vi "从数据库获取数据通用可配置(子VI).vi"(8 "错误输入（无错误）":errorcluster, 9 "查询参数数组":string[](array[string])=["CODMn", "CODCr", "DO", "铜", "PH", "氨氮", "比电导率", "水温", "COD", "浊度", "总氮", "总磷", "叶绿素a", "藻密度", "水位", "流速", "瞬时流量", "累积流量", "亚硝酸盐", "硫化物", "ORP", "铅", "镉", "锌", "镍", "锰", "汞"], 10 "table输入":string="实时数据") -> (0 "错误输出":errorcluster, 3 "簇数组":cluster{"待发送数据":string[][]}[][](array[cluster]))   [LabVIEW 2016, in "数据传输系统-02.lvlib"]
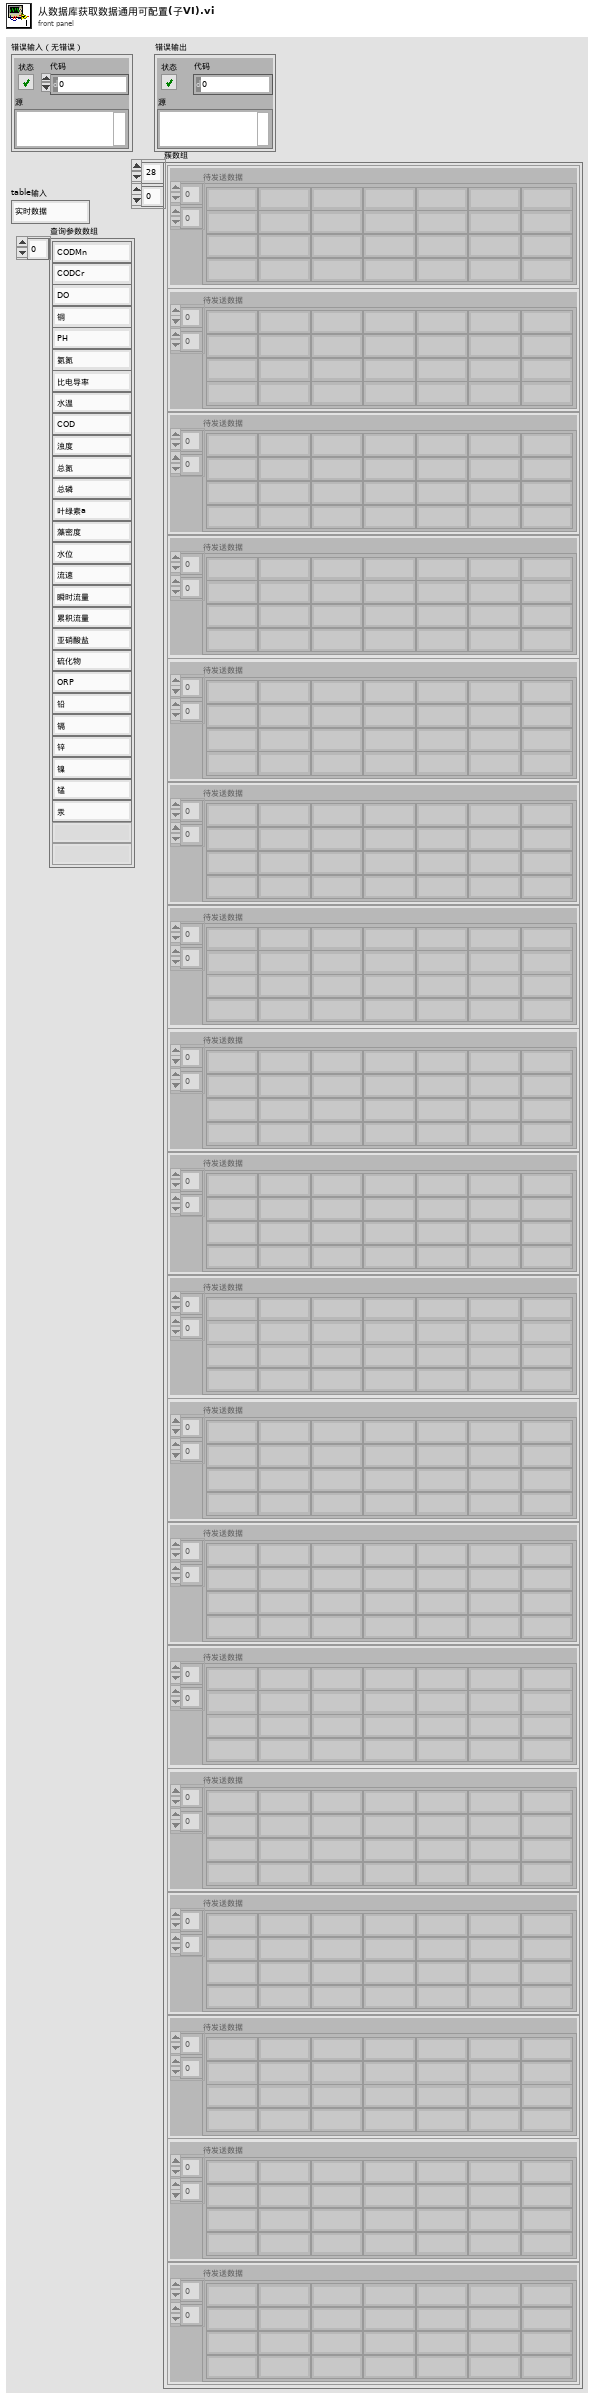
[diagram p1: front panel]
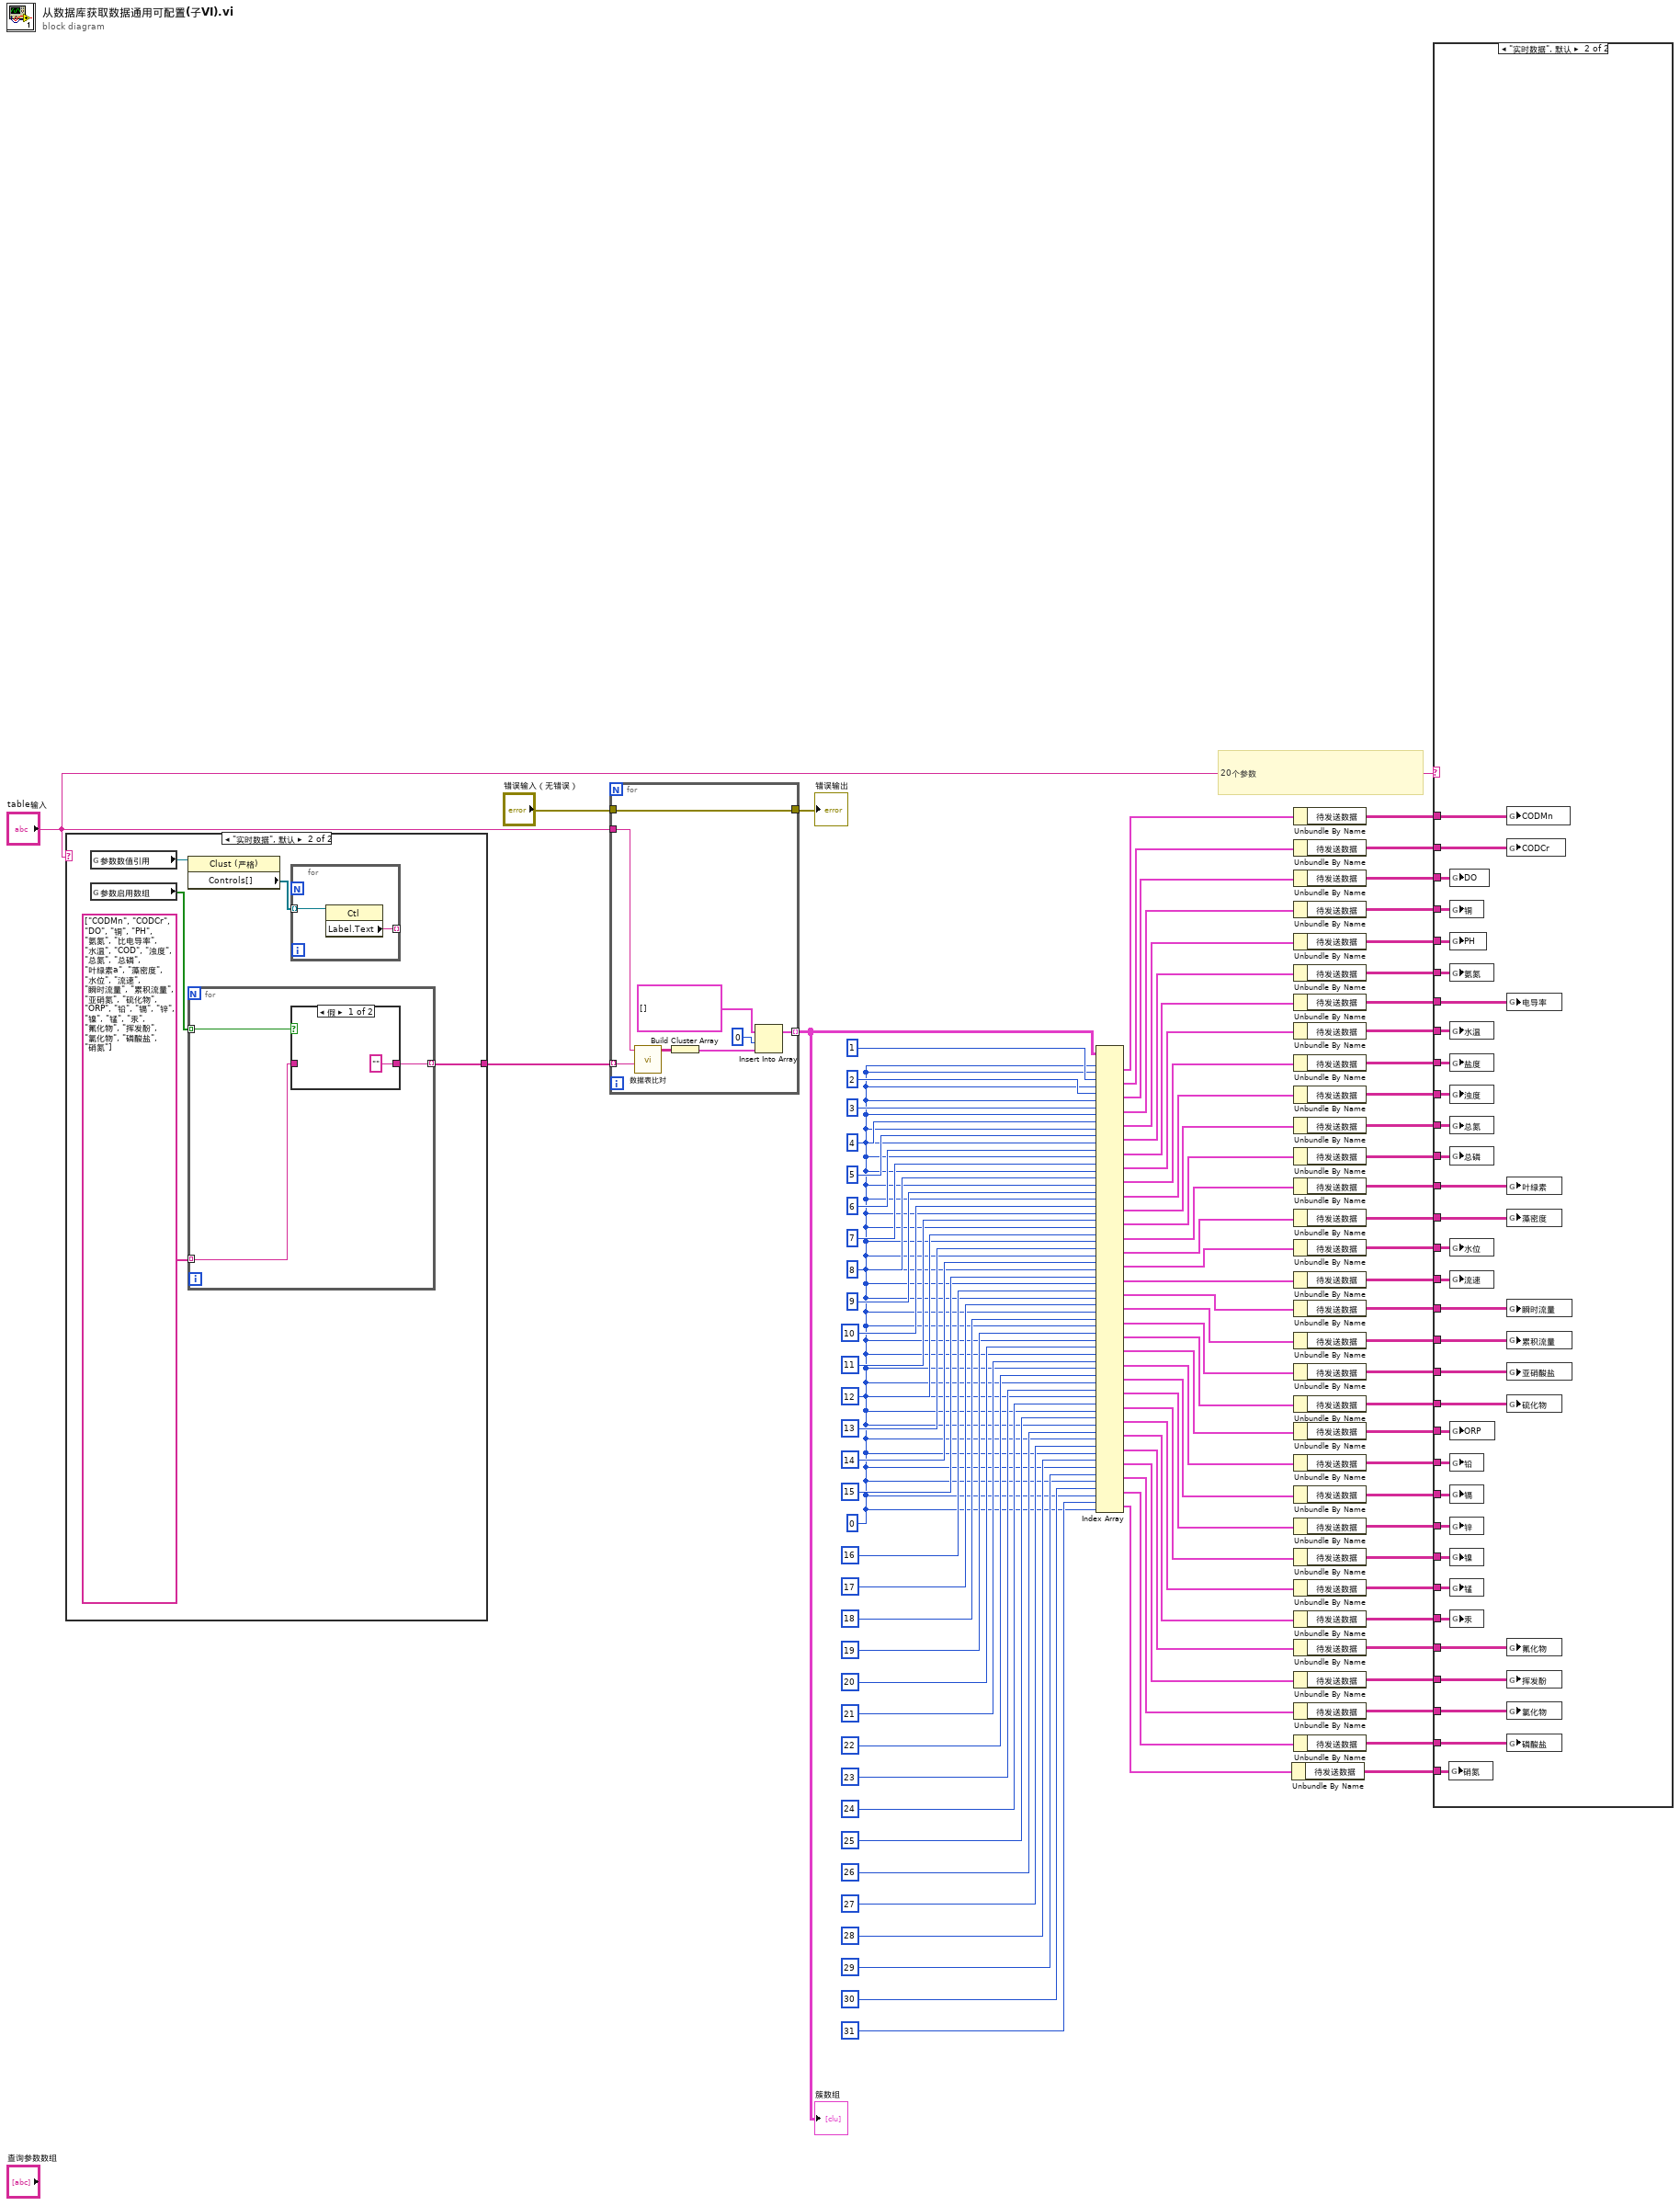
[diagram p0: block diagram]
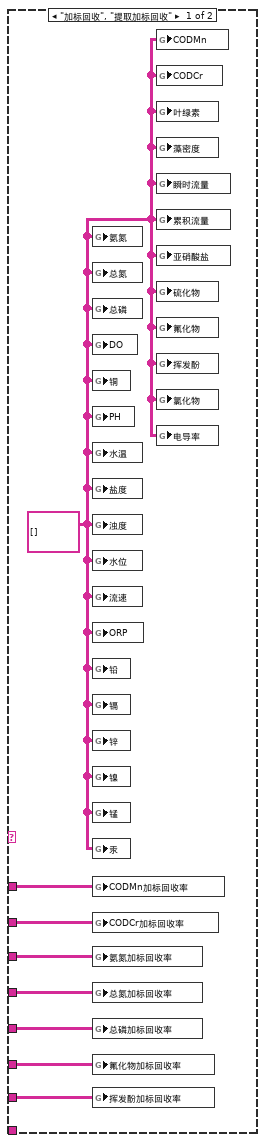
[diagram p2: hidden frame]
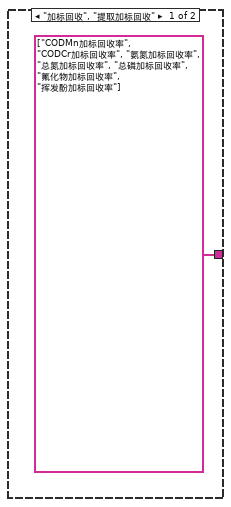
[diagram p3: hidden frame]
diagram:
  w5 = 0 ("索引 (行)")
  # "20个参数"
  n1 = case shown="\"实时数据\", 默认" "table输入" {
    tunnel: [string[] ["CODMn加标回收率", "CODCr加标回收率", "氨氮加标回收率", "总氮加标回收率", "总磷加标回收率", "氟化物加标回收率", "挥发酚加标回收率"] ("查询参数数组") w106] -> w58
    frame "加标回收", "提取加标回收" {
    }
    frame "实时数据", Default {
      n2 = global read "断电保存全局.vi" "参数数值引用"() -> (w105:refnum<vi>)
      n3 = global read "断电保存全局.vi" "参数启用数组"() -> (w107:bool[])
      n4 = property class="Clust (严格)"(reference=w105) -> ("Controls[]"=w104:refnum<vi>[])  [unwired: 1 in, 2 out]
      n5 = for {
        tunnel: w107 -> [w112] mode=indexing
        tunnel: string[] ["CODMn", "CODCr", "DO", "铜", "PH", "氨氮", "比电导率", "水温", "COD", "浊度", "总氮", "总磷", "叶绿素a", "藻密度", "水位", "流速", "瞬时流量", "累积流量", "亚硝氮", "硫化物", "ORP", "铅", "镉", "锌", "镍", "锰", "汞", "氟化物", "挥发酚", "氯化物", "磷酸盐", "硝氮"] ("数组") -> [w111] mode=indexing
        tunnel: [w110] -> w106 mode=indexing
        n6 = case shown="假" w112 {
          tunnel: ["" w114] -> w110
          tunnel: w111 -> [_ w114]
          frame False {
          }
          frame True {
          }
        }
      }
      n7 = for {
        tunnel: w104 -> [w109] mode=indexing
        tunnel: [w108] -> _ mode=indexing
        n8 = property class="Ctl"(reference=w109) -> ("Label.Text"=w108:string)  [unwired: 1 in, 2 out]
      }
    }
  }
  n9 = for {
    tunnel: w58 -> [w116] mode=indexing
    tunnel: [w120] -> w100 mode=indexing
    tunnel: "table输入" -> [w117]
    tunnel: [w115] -> w101
    tunnel: "错误输入（无错误）" -> [w115]
    n10 = call "数据表比对.vi"("查询元素输入"=w116, "table输入"=w117) -> ("待发送数据"=w122:string[][])  [unwired: 6 in, 3 out]
    n11 = Build Cluster Array(w122) -> (w121:cluster{"待发送数据":string[][]}[])
    n12 = Insert Into Array(array=cluster{"待发送数据":string[][]}[] [] ("簇数组"), index=0 ("索引"), new element=w121) -> (w120:cluster{"待发送数据":string[][]}[])
  }
  "簇数组" <- w100
  "错误输出" <- w101
  n13 = Index Array(array=w100, index (row) #1=w5, index (col) #1=w5, index (row) #2=1 ("索引 (行)"), index (col) #2=w5, index (row) #3=2 ("索引 (行)"), index (col) #3=w5, index (row) #4=3 ("索引 (行)"), index (col) #4=w5, index (row) #5=4 ("索引 (行)"), index (col) #5=w5, index (row) #6=5 ("索引 (行)"), index (col) #6=w5, index (row) #7=6 ("索引 (行)"), index (col) #7=w5, index (row) #8=7 ("索引 (行)"), index (col) #8=w5, index (row) #9=8 ("索引 (行)"), index (col) #9=w5, index (row) #10=9 ("索引 (行)"), index (col) #10=w5, index (row) #11=10 ("索引 (行)"), index (col) #11=w5, index (row) #12=11 ("索引 (行)"), index (col) #12=w5, index (row) #13=12 ("索引 (行)"), index (col) #13=w5, index (row) #14=13 ("索引 (行)"), index (col) #14=w5, index (row) #15=14 ("禁用的索引 (行)"), index (col) #15=w5, index (row) #16=15 ("禁用的索引 (行)"), index (col) #16=w5, index (row) #17=16 ("禁用的索引 (行)"), index (col) #17=w5, index (row) #18=17 ("禁用的索引 (行)"), index (col) #18=w5, index (row) #19=18 ("禁用的索引 (行)"), index (col) #19=w5, index (row) #20=19 ("禁用的索引 (行)"), index (col) #20=w5, index (row) #21=20 ("禁用的索引 (行)"), index (col) #21=w5, index (row) #22=21 ("禁用的索引 (行)"), index (col) #22=w5, index (row) #23=22 ("禁用的索引 (行)"), index (col) #23=w5, index (row) #24=23 ("禁用的索引 (行)"), index (col) #24=w5, index (row) #25=24 ("禁用的索引 (行)"), index (col) #25=w5, index (row) #26=25 ("禁用的索引 (行)"), index (col) #26=w5, index (row) #27=26 ("禁用的索引 (行)"), index (col) #27=w5, index (row) #28=27 ("禁用的索引 (行)"), index (col) #28=w5, index (row) #29=28 ("禁用的索引 (行)"), index (col) #29=w5, index (row) #30=29 ("禁用的索引 (行)"), index (col) #30=w5, index (row) #31=30 ("索引 (行)"), index (col) #31=w5, index (row) #32=31 ("索引 (行)"), index (col) #32=w5) -> (element #1=w99:cluster{"待发送数据":string[][]}, element #2=w84:cluster{"待发送数据":string[][]}, element #3=w83:cluster{"待发送数据":string[][]}, element #4=w82:cluster{"待发送数据":string[][]}, element #5=w81:cluster{"待发送数据":string[][]}, element #6=w80:cluster{"待发送数据":string[][]}, element #7=w78:cluster{"待发送数据":string[][]}, element #8=w79:cluster{"待发送数据":string[][]}, element #9=w77:cluster{"待发送数据":string[][]}, element #10=w76:cluster{"待发送数据":string[][]}, element #11=w75:cluster{"待发送数据":string[][]}, element #12=w74:cluster{"待发送数据":string[][]}, element #13=w73:cluster{"待发送数据":string[][]}, element #14=w72:cluster{"待发送数据":string[][]}, element #15=w53:cluster{"待发送数据":string[][]}, element #16=w51:cluster{"待发送数据":string[][]}, element #17=w50:cluster{"待发送数据":string[][]}, element #18=w49:cluster{"待发送数据":string[][]}, element #19=w44:cluster{"待发送数据":string[][]}, element #20=w40:cluster{"待发送数据":string[][]}, element #21=w39:cluster{"待发送数据":string[][]}, element #22=w32:cluster{"待发送数据":string[][]}, element #23=w31:cluster{"待发送数据":string[][]}, element #24=w30:cluster{"待发送数据":string[][]}, element #25=w24:cluster{"待发送数据":string[][]}, element #26=w22:cluster{"待发送数据":string[][]}, element #27=w21:cluster{"待发送数据":string[][]}, element #28=w16:cluster{"待发送数据":string[][]}, element #29=w11:cluster{"待发送数据":string[][]}, element #30=w10:cluster{"待发送数据":string[][]}, element #31=w4:cluster{"待发送数据":string[][]}, element #32=w1:cluster{"待发送数据":string[][]})
  n14 = Unbundle By Name(w1) -> ("待发送数据"=w2:string[][])
  n15 = Unbundle By Name(w99) -> ("待发送数据"=w98:string[][])
  n16 = Unbundle By Name(w84) -> ("待发送数据"=w71:string[][])
  n17 = Unbundle By Name(w83) -> ("待发送数据"=w70:string[][])
  n18 = Unbundle By Name(w82) -> ("待发送数据"=w69:string[][])
  n19 = Unbundle By Name(w81) -> ("待发送数据"=w68:string[][])
  n20 = Unbundle By Name(w80) -> ("待发送数据"=w67:string[][])
  n21 = Unbundle By Name(w78) -> ("待发送数据"=w66:string[][])
  n22 = Unbundle By Name(w79) -> ("待发送数据"=w65:string[][])
  n23 = Unbundle By Name(w77) -> ("待发送数据"=w64:string[][])
  n24 = Unbundle By Name(w76) -> ("待发送数据"=w63:string[][])
  n25 = Unbundle By Name(w75) -> ("待发送数据"=w62:string[][])
  n26 = Unbundle By Name(w74) -> ("待发送数据"=w61:string[][])
  n27 = Unbundle By Name(w73) -> ("待发送数据"=w59:string[][])
  n28 = Unbundle By Name(w72) -> ("待发送数据"=w60:string[][])
  n29 = Unbundle By Name(w53) -> ("待发送数据"=w52:string[][])
  n30 = Unbundle By Name(w51) -> ("待发送数据"=w48:string[][])
  n31 = Unbundle By Name(w50) -> ("待发送数据"=w47:string[][])
  n32 = Unbundle By Name(w49) -> ("待发送数据"=w46:string[][])
  n33 = Unbundle By Name(w44) -> ("待发送数据"=w38:string[][])
  n34 = Unbundle By Name(w40) -> ("待发送数据"=w37:string[][])
  n35 = Unbundle By Name(w39) -> ("待发送数据"=w36:string[][])
  n36 = Unbundle By Name(w32) -> ("待发送数据"=w29:string[][])
  n37 = Unbundle By Name(w31) -> ("待发送数据"=w28:string[][])
  n38 = Unbundle By Name(w30) -> ("待发送数据"=w27:string[][])
  n39 = Unbundle By Name(w24) -> ("待发送数据"=w23:string[][])
  n40 = Unbundle By Name(w22) -> ("待发送数据"=w20:string[][])
  n41 = Unbundle By Name(w21) -> ("待发送数据"=w19:string[][])
  n42 = Unbundle By Name(w16) -> ("待发送数据"=w15:string[][])
  n43 = Unbundle By Name(w11) -> ("待发送数据"=w9:string[][])
  n44 = Unbundle By Name(w10) -> ("待发送数据"=w8:string[][])
  n45 = Unbundle By Name(w4) -> ("待发送数据"=w3:string[][])
  n46 = case shown="\"实时数据\", 默认" "table输入" {
    tunnel: w98 -> [w130 w162]
    tunnel: w71 -> [w129 w161]
    tunnel: w70 -> [w128 w160]
    tunnel: w69 -> [w127 w159]
    tunnel: w68 -> [w126 w158]
    tunnel: w67 -> [w125 w157]
    tunnel: w66 -> [w124 w156]
    tunnel: w65 -> [_ w155]
    tunnel: w64 -> [_ w154]
    tunnel: w63 -> [_ w153]
    tunnel: w62 -> [_ w152]
    tunnel: w61 -> [_ w151]
    tunnel: w60 -> [_ w150]
    tunnel: w59 -> [_ w149]
    tunnel: w52 -> [_ w148]
    tunnel: w48 -> [_ w147]
    tunnel: w47 -> [_ w146]
    tunnel: w46 -> [_ w145]
    tunnel: w38 -> [_ w144]
    tunnel: w37 -> [_ w143]
    tunnel: w36 -> [_ w142]
    tunnel: w29 -> [_ w141]
    tunnel: w28 -> [_ w140]
    tunnel: w27 -> [_ w139]
    tunnel: w23 -> [_ w138]
    tunnel: w20 -> [_ w137]
    tunnel: w19 -> [_ w136]
    tunnel: w15 -> [_ w135]
    tunnel: w9 -> [_ w134]
    tunnel: w8 -> [_ w133]
    tunnel: w3 -> [_ w132]
    tunnel: w2 -> [_ w131]
    frame "加标回收", "提取加标回收" {
      w123 = string[][] [] ("DO")
      n47 = global write "全局 所有参数.vi" "氨氮"(w123) -> ()
      n48 = global write "全局 所有参数.vi" "总氮"(w123) -> ()
      n49 = global write "全局 所有参数.vi" "总磷"(w123) -> ()
      n50 = global write "全局 所有参数.vi" "DO"(w123) -> ()
      n51 = global write "全局 所有参数.vi" "铜"(w123) -> ()
      n52 = global write "全局 所有参数.vi" "PH"(w123) -> ()
      n53 = global write "全局 所有参数.vi" "水温"(w123) -> ()
      n54 = global write "全局 所有参数.vi" "盐度"(w123) -> ()
      n55 = global write "全局 所有参数.vi" "浊度"(w123) -> ()
      n56 = global write "全局 所有参数.vi" "水位"(w123) -> ()
      n57 = global write "全局 所有参数.vi" "流速"(w123) -> ()
      n58 = global write "全局 所有参数.vi" "ORP"(w123) -> ()
      n59 = global write "全局 所有参数.vi" "铅"(w123) -> ()
      n60 = global write "全局 所有参数.vi" "镉"(w123) -> ()
      n61 = global write "全局 所有参数.vi" "锌"(w123) -> ()
      n62 = global write "全局 所有参数.vi" "镍"(w123) -> ()
      n63 = global write "全局 所有参数.vi" "锰"(w123) -> ()
      n64 = global write "全局 所有参数.vi" "汞"(w123) -> ()
      n65 = global write "全局 所有参数.vi" "CODMn加标回收率"(w130) -> ()
      n66 = global write "全局 所有参数.vi" "CODCr加标回收率"(w129) -> ()
      n67 = global write "全局 所有参数.vi" "氨氮加标回收率"(w128) -> ()
      n68 = global write "全局 所有参数.vi" "总氮加标回收率"(w127) -> ()
      n69 = global write "全局 所有参数.vi" "总磷加标回收率"(w126) -> ()
      n70 = global write "全局 所有参数.vi" "氟化物加标回收率"(w125) -> ()
      n71 = global write "全局 所有参数.vi" "挥发酚加标回收率"(w124) -> ()
      n72 = global write "全局 所有参数.vi" "CODMn"(w123) -> ()
      n73 = global write "全局 所有参数.vi" "CODCr"(w123) -> ()
      n74 = global write "全局 所有参数.vi" "叶绿素"(w123) -> ()
      n75 = global write "全局 所有参数.vi" "藻密度"(w123) -> ()
      n76 = global write "全局 所有参数.vi" "瞬时流量"(w123) -> ()
      n77 = global write "全局 所有参数.vi" "累积流量"(w123) -> ()
      n78 = global write "全局 所有参数.vi" "亚硝酸盐"(w123) -> ()
      n79 = global write "全局 所有参数.vi" "硫化物"(w123) -> ()
      n80 = global write "全局 所有参数.vi" "氟化物"(w123) -> ()
      n81 = global write "全局 所有参数.vi" "挥发酚"(w123) -> ()
      n82 = global write "全局 所有参数.vi" "氯化物"(w123) -> ()
      n83 = global write "全局 所有参数.vi" "电导率"(w123) -> ()
    }
    frame "实时数据", Default {
      n84 = global write "全局 所有参数.vi" "硝氮"(w131) -> ()
      n85 = global write "全局 所有参数.vi" "DO"(w160) -> ()
      n86 = global write "全局 所有参数.vi" "铜"(w159) -> ()
      n87 = global write "全局 所有参数.vi" "PH"(w158) -> ()
      n88 = global write "全局 所有参数.vi" "氨氮"(w157) -> ()
      n89 = global write "全局 所有参数.vi" "水温"(w155) -> ()
      n90 = global write "全局 所有参数.vi" "盐度"(w154) -> ()
      n91 = global write "全局 所有参数.vi" "浊度"(w153) -> ()
      n92 = global write "全局 所有参数.vi" "总氮"(w152) -> ()
      n93 = global write "全局 所有参数.vi" "总磷"(w151) -> ()
      n94 = global write "全局 所有参数.vi" "水位"(w148) -> ()
      n95 = global write "全局 所有参数.vi" "流速"(w147) -> ()
      n96 = global write "全局 所有参数.vi" "ORP"(w142) -> ()
      n97 = global write "全局 所有参数.vi" "铅"(w141) -> ()
      n98 = global write "全局 所有参数.vi" "镉"(w140) -> ()
      n99 = global write "全局 所有参数.vi" "锌"(w139) -> ()
      n100 = global write "全局 所有参数.vi" "镍"(w138) -> ()
      n101 = global write "全局 所有参数.vi" "锰"(w137) -> ()
      n102 = global write "全局 所有参数.vi" "汞"(w136) -> ()
      n103 = global write "全局 所有参数.vi" "CODMn"(w162) -> ()
      n104 = global write "全局 所有参数.vi" "CODCr"(w161) -> ()
      n105 = global write "全局 所有参数.vi" "电导率"(w156) -> ()
      n106 = global write "全局 所有参数.vi" "叶绿素"(w149) -> ()
      n107 = global write "全局 所有参数.vi" "藻密度"(w150) -> ()
      n108 = global write "全局 所有参数.vi" "瞬时流量"(w146) -> ()
      n109 = global write "全局 所有参数.vi" "累积流量"(w145) -> ()
      n110 = global write "全局 所有参数.vi" "亚硝酸盐"(w144) -> ()
      n111 = global write "全局 所有参数.vi" "硫化物"(w143) -> ()
      n112 = global write "全局 所有参数.vi" "氟化物"(w135) -> ()
      n113 = global write "全局 所有参数.vi" "挥发酚"(w134) -> ()
      n114 = global write "全局 所有参数.vi" "氯化物"(w133) -> ()
      n115 = global write "全局 所有参数.vi" "磷酸盐"(w132) -> ()
    }
  }
